vi "test14.1-MappingRelationshipByExternalRegistration_API_State.vi"(8 "error in (no error)":errorcluster, 11 "TestCase in":refnum<class "testcase-CSMBroadcast.lvclass">) -> (0 "error out":errorcluster, 3 "TestCase out":refnum<class "testcase-CSMBroadcast.lvclass">)   [LabVIEW 2017, in "testcase-CSMBroadcast.lvclass"]
uses:
  testcase-CSMBroadcast.lvclass
  src/user.lib/_NEVSTOP/Communicable State Machine(CSM)/Communicable State Machine.lvlib
  <vilib>/addons/_JKI Toolkits/VI Tester/TestCase.llb/TestCase.lvclass
  CSM/CSM-Testcase.lvlib
  C:/Program Files (x86)/National Instruments/LabVIEW 2017/vi.lib/addons/_JKI Toolkits/VI Tester/TestCase.llb/TestCase.lvclass
panel:
  out "Loop Count":i32
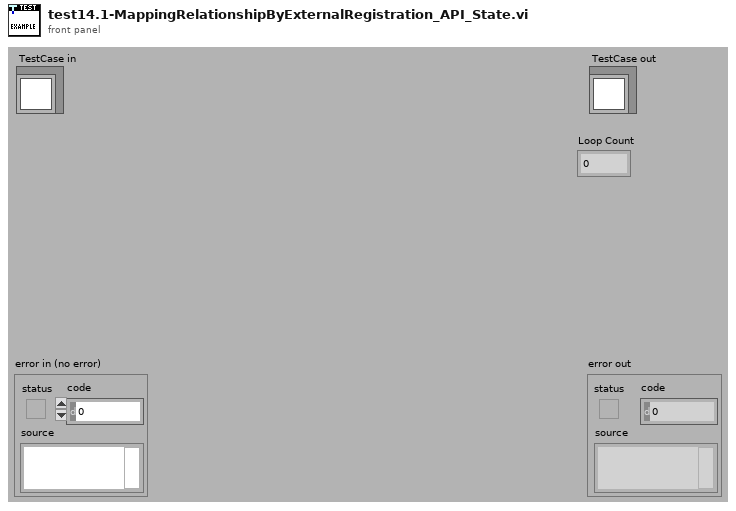
[diagram p1: front panel]
types:
  T1 = cluster{"Status":string, "Source CSM":string, "Target CSM":string, "Target API":string}[]
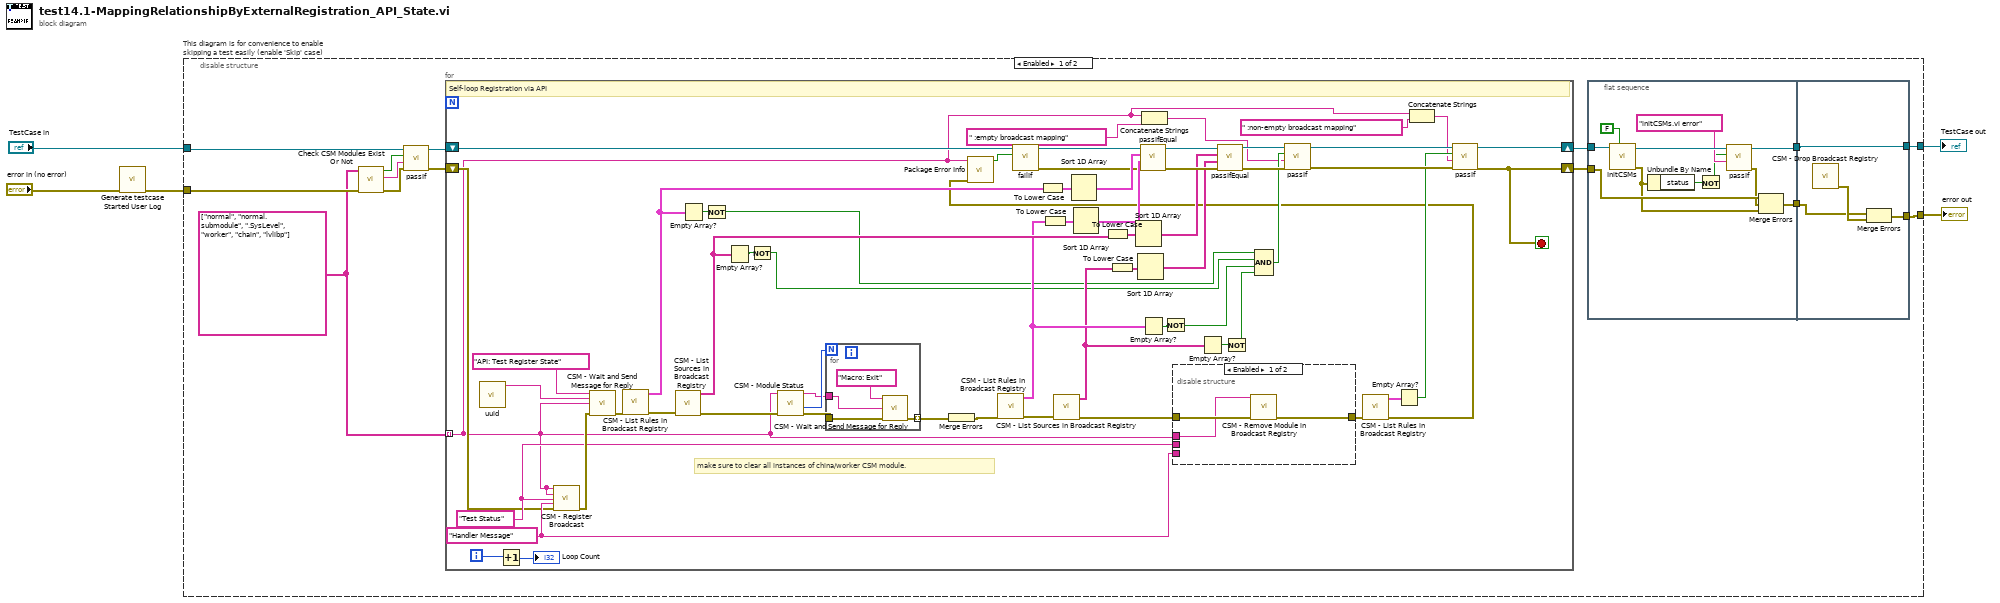
[diagram p0: block diagram]
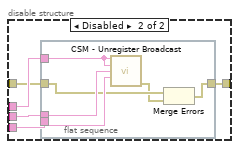
[diagram p2: hidden frame]
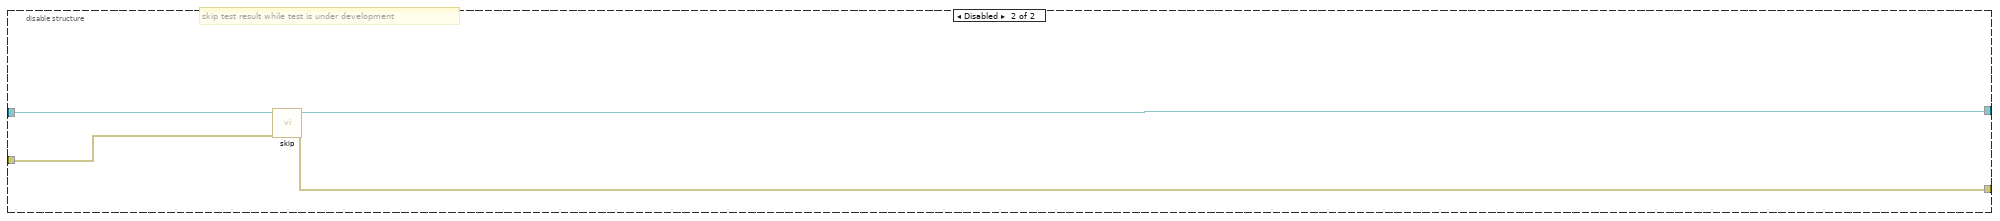
[diagram p3: hidden frame]
diagram:
  n1 = call "Generate testcase Started User Log.vi"("Error In"="error in (no error)") -> ("error out"=w1:errorcluster)  [unwired: 10 in]
  n2 = disable-structure "This diagram is for convenience to enable skipping a test easily (enable 'Skip' case)" shown="Enabled" {
    disable-tunnel: "TestCase in" -> [w16 w116]
    disable-tunnel: [w7 w114] -> w2
    disable-tunnel: [w6 w115] -> w4
    disable-tunnel: w1 -> [w13 w113]
    frame Enabled {
      w12 = string[] ["normal", "normal.submodule", ".SysLevel", "worker", "chain", "lvlibp"]
      n3 = call "Check CSM Modules Exist Or Not.vi"("error in"=w13, "CSM names in"=w12) -> ("error out"=w17:errorcluster, "Debug string"=w18:string, "All Modules Exist?"=w19:bool)  [unwired: 7 in]
      n4 = call-dynamic "passIf.vi"("error in (no error)"=w17, "message (\"\")"=w18, "pass"=w19, "TestCase in"=w16) -> ("error out"=w14:errorcluster, "TestCase out"=w15:refnum<class "testcase-CSMBroadcast.lvclass">)  [unwired: 6 in]
      n5 = for {
        tunnel: w12 -> [w38] mode=indexing
        shift-right: [w54] -> w9
        shift-left: w15 -> [w43]
        shift-right: [w49] -> w8
        shift-left: w14 -> [w50]
        i -> [w77]
        stop <- w49 stop-if-true
        w58 = "Handler Message" ("Response Message (If \"\", Same as Source Message)")
        w57 = "Test Status" ("Status")
        # "make sure to clear all instances of china/worker CSM module."
        # "Self-loop Registration via API"
        n6 = call "uuid.vi"() -> ("UUID"=w93:string)  [unwired: 11 in]
        n7 = Increment(x=w77) -> (x+1=→"Loop Count":i32)
        n8 = call "CSM - Register Broadcast.vi"("CSM Name(Empty for Broadcast Event)"=w38, "Source CSM Name (* as Default)"=w38, "Trigger"=w57, "API (If \"\", Same as Trigger)"=w58, "Error In"=w50) -> ("error out"=w60:errorcluster)  [unwired: 9 in, 1 out]
        n9 = call "CSM - Wait and Send Message for Reply.vi"("State"="API: Test Register State", "Arguments (\"\")"=w93, "Target Module"=w38, "Error In (No Error)"=w60) -> ("error out"=w92:errorcluster)  [unwired: 8 in, 3 out]
        n10 = call "CSM - List Rules in Broadcast Registry.vi"("error in (no error)"=w92) -> ("error out"=w89:errorcluster, "Rule Entries"=w75:T1)  [unwired: 8 in, 1 out]
        n11 = call "CSM - List Sources in Broadcast Registry.vi"("error in (no error)"=w89) -> ("error out"=w45:errorcluster, "Broadcast Names"=w72:string[])  [unwired: 9 in]
        n12 = Empty Array?(array=w75) -> (empty?=w74:bool)
        n13 = Not(x=w74) -> (.not. x?=w67:bool)
        n14 = Empty Array?(array=w72) -> (empty?=w73:bool)
        n15 = Not(x=w73) -> (.not. x?=w66:bool)
        n16 = call "CSM - Module Status.vi"("Error In"=w45, "CSM Name"=w38) -> ("error out"=w46:errorcluster, "#Nodes"=w48:i32, "CSM Name (Dup)"=w47:string)  [unwired: 5 in, 2 out]
        n17 = for {
          N: w48 -> [_]
          tunnel: w47 -> [w96]
          tunnel: w46 -> [w95]
          tunnel: [w97] -> w91 mode=indexing
          n18 = call "CSM - Wait and Send Message for Reply.vi"("State"="Macro: Exit", "Target Module"=w96, "Error In (No Error)"=w95) -> ("error out"=w97:errorcluster)  [unwired: 9 in, 3 out]
        }
        n19 = Merge Errors(w91) -> (w90:errorcluster)
        n20 = call "CSM - List Rules in Broadcast Registry.vi"("error in (no error)"=w90) -> ("error out"=w88:errorcluster, "Rule Entries"=w70:T1)  [unwired: 8 in, 1 out]
        n21 = To Lower Case(string=w75) -> (all lower case string=w87:T1)
        n22 = To Lower Case(string=w70) -> (all lower case string=w86:T1)
        n23 = call "CSM - List Sources in Broadcast Registry.vi"("error in (no error)"=w88) -> ("error out"=w59:errorcluster, "Broadcast Names"=w68:string[])  [unwired: 9 in]
        n24 = Sort 1D Array(array=w87) -> (sorted array=w85:T1)
        n25 = Sort 1D Array(array=w86) -> (sorted array=w84:T1)
        n26 = To Lower Case(string=w72) -> (all lower case string=w81:string[])
        n27 = To Lower Case(string=w68) -> (all lower case string=w80:string[])
        n28 = Sort 1D Array(array=w81) -> (sorted array=w79:string[])
        n29 = Sort 1D Array(array=w80) -> (sorted array=w78:string[])
        n30 = Empty Array?(array=w70) -> (empty?=w71:bool)
        n31 = Concatenate Strings(w38, " :empty broadcast mapping" ("string")) -> (w36:string)
        n32 = Not(x=w71) -> (.not. x?=w65:bool)
        n33 = disable-structure shown="Enabled" {
          disable-tunnel: w59 -> [w101 w103]
          disable-tunnel: [w100 w102] -> w56
          disable-tunnel: w38 -> [w99 w104]
          disable-tunnel: w57 -> [_ w106]
          disable-tunnel: w58 -> [_ w105]
          frame Enabled {
            n34 = call "CSM - Remove Module in Broadcast Registry.vi"("CSM Name"=w99, "Error In"=w101) -> ("error out"=w100:errorcluster)  [unwired: 12 in, 1 out]
          }
          frame Disabled {
            n35 = flat-sequence {
              tunnel: w106 -> [w112]
              tunnel: w105 -> [w111]
              tunnel: w104 -> [w110]
              tunnel: w103 -> [w109]
              tunnel: [w107] -> w102
              frame #0 {
                n36 = call "CSM - Unregister Broadcast.vi"("CSM Name(Empty for Broadcast Event)"=w110, "Source CSM Name (* as Default)"=w110, "Trigger"=w112, "API (\"*\" as Default)"=w111) -> ("error out"=w108:errorcluster)  [unwired: 10 in, 1 out]
                n37 = Merge Errors(w109, w108) -> (w107:errorcluster)
              }
            }
          }
        }
        n38 = Empty Array?(array=w68) -> (empty?=w69:bool)
        n39 = Not(x=w69) -> (.not. x?=w64:bool)
        n40 = Compound Arithmetic op=AND(w67, w66, w65, w64) -> (w61:bool)
        n41 = call "CSM - List Rules in Broadcast Registry.vi"("error in (no error)"=w56) -> ("error out"=w40:errorcluster, "Rule Entries"=w52:T1)  [unwired: 8 in, 1 out]
        n42 = call "Package Error Info.vi"("error in"=w40, "String in"=w38) -> ("error status"=w44:bool)  [unwired: 8 in, 1 out]
        n43 = call-dynamic "failIf.vi"("fail"=w44, "TestCase in"=w43) -> ("error out"=w41:errorcluster, "TestCase out"=w42:refnum<class "testcase-CSMBroadcast.lvclass">)  [unwired: 8 in]
        n44 = call-dynamic "passIfEqual.vi"("error in (no error)"=w41, "y"=w84, "x"=w85, "TestCase in"=w42) -> ("error out"=w82:errorcluster, "TestCase out"=w83:refnum<class "testcase-CSMBroadcast.lvclass">)  [unwired: 6 in]
        n45 = call-dynamic "passIfEqual.vi"("error in (no error)"=w82, "y"=w78, "x"=w79, "TestCase in"=w83) -> ("error out"=w62:errorcluster, "TestCase out"=w63:refnum<class "testcase-CSMBroadcast.lvclass">)  [unwired: 6 in]
        n46 = call-dynamic "passIf.vi"("error in (no error)"=w62, "message (\"\")"=w36, "pass"=w61, "TestCase in"=w63) -> ("error out"=w53:errorcluster, "TestCase out"=w55:refnum<class "testcase-CSMBroadcast.lvclass">)  [unwired: 6 in]
        n47 = Empty Array?(array=w52) -> (empty?=w51:bool)
        n48 = Concatenate Strings(w38, " :non-empty broadcast mapping" ("string")) -> (w35:string)
        n49 = call-dynamic "passIf.vi"("error in (no error)"=w53, "message (\"\")"=w35, "pass"=w51, "TestCase in"=w55) -> ("error out"=w49:errorcluster, "TestCase out"=w54:refnum<class "testcase-CSMBroadcast.lvclass">)  [unwired: 6 in]
      }
      n50 = flat-sequence {
        tunnel: w9 -> [w30]
        tunnel: [w27] -> w11
        tunnel: w8 -> [w24]
        tunnel: [w21] -> w10
        tunnel: w11 -> [w33]
        tunnel: [w33] -> w7
        tunnel: [w32] -> w6
        tunnel: w10 -> [w31]
        frame #0 {
          n51 = call "InitCSMs.vi"("Enable building lvlibp?"=FALSE, "testcase-CSMStatus in"=w30) -> ("error out"=w22:errorcluster, "testcase-CSMStatus out"=w28:refnum<class "testcase-CSMBroadcast.lvclass">)  [unwired: 8 in]
          n52 = Unbundle By Name(w22) -> ("status"=w26:bool)
          n53 = Not(x=w26) -> (.not. x?=w20:bool)
          n54 = call-dynamic "passIf.vi"("message (\"\")"="initCSMs.vi error" ("message (\"\")"), "pass"=w20, "TestCase in"=w28) -> ("error out"=w23:errorcluster, "TestCase out"=w27:refnum<class "testcase-CSMBroadcast.lvclass">)  [unwired: 7 in]
          n55 = Merge Errors(w24, w23, w22) -> (w21:errorcluster)
        }
        frame #1 {
          n56 = call "CSM - Drop Broadcast Registry.vi"() -> ("error out"=w34:errorcluster)  [unwired: 15 in]
          n57 = Merge Errors(w31, w34) -> (w32:errorcluster)
        }
      }
    }
    frame Disabled {
      # "skip test result while test is under development"
      n58 = call <vilib>:"skip.vi"("error in (no error)"=w113, "TestCase in"=w116) -> ("error out"=w115:errorcluster, "TestCase out"=w114:refnum<class "testcase-CSMBroadcast.lvclass">)  [unwired: 8 in]
    }
  }
  "error out" <- w4
  "TestCase out" <- w2
